vi "Whitespace_to_Zeros.vi"(2 "Input String":string) -> (6 "Output String":string)   [LabVIEW 2011]
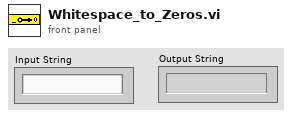
[diagram p1: front panel]
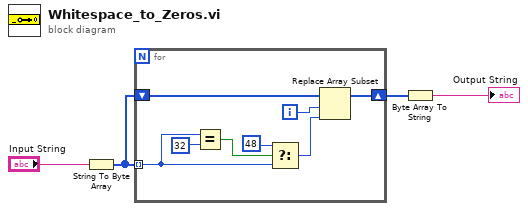
[diagram p0: block diagram]
diagram:
  n1 = String To Byte Array(string="Input String") -> (unsigned byte array=w3:u8[])
  n2 = for {
    tunnel: w3 -> [w8] mode=indexing
    shift-right: [w5] -> w2
    shift-left: w3 -> [w11]
    i -> [w6]
    n3 = Equal?(x=w8, y=u8 32) -> (x = y?=w10:bool)
    n4 = Select(t=u8 48 ("y"), s=w10, f=w8) -> (s? t:f=w7:u8)
    n5 = Replace Array Subset(array=w11, new element=w7, index=w6) -> (w5:u8[])
  }
  n6 = Byte Array To String(unsigned byte array=w2) -> (string=→"Output String":string)
